vi "Create.vi"(8 "error in (no error)":errorcluster, 10 "Input":string) -> (0 "error out":errorcluster, 3 "Proto":refnum<class "NetAn.lvclass">)   [LabVIEW 2020, in "NetAn.lvclass"]
uses:
  NetAn.lvclass
  <vilib>/Utility/miscctls.llb/LVMapReplaceAction.ctl
  NetAn.lvclass/NetAn.ctl
  Global 1.vi
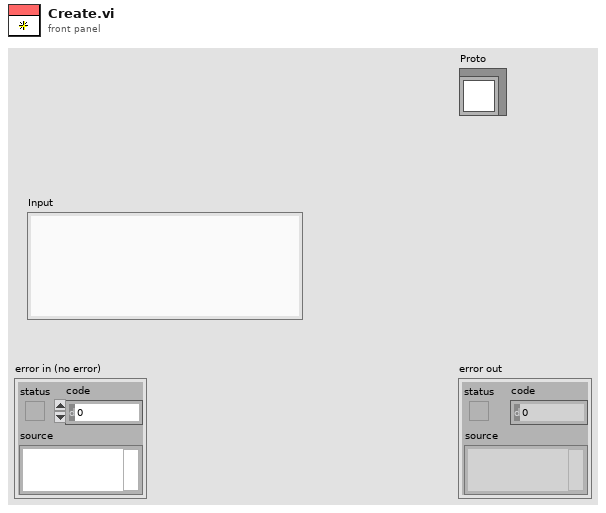
[diagram p1: front panel]
types:
  T1 = typedef "LVMapReplaceAction.ctl" = enum32{"Modify Entry only if found", "Add or Modify Entry", "Delete Entry"}
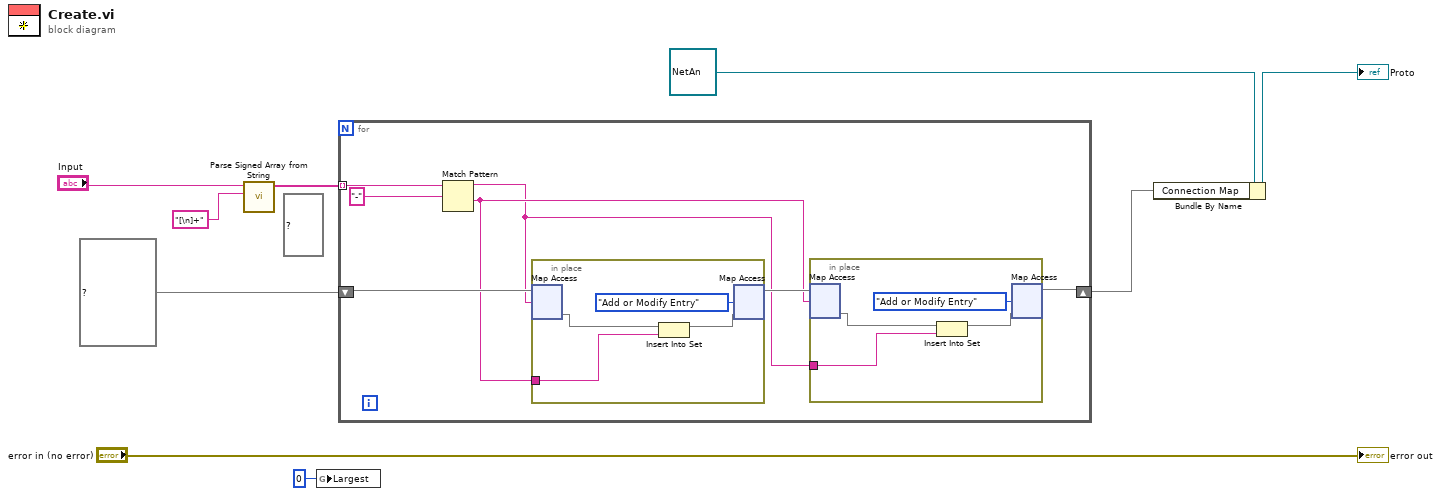
[diagram p0: block diagram]
diagram:
  (unwired) set{string} {} ("set in")
  n1 = call "Parse Signed Array from String.vi"("Delimiter regex"="[\n]+", "Input"="Input") -> ("Parsed Array"=w4:string[])  [unwired: 8 in, 1 out]
  n2 = global write "Global 1.vi" "Largest"(0 ("Largest")) -> ()
  n3 = for {
    tunnel: w4 -> [w16] mode=indexing
    shift-right: [w12] -> w2
    shift-left: map{string, set{string}} {} ("map") -> [w14]
    n4 = Match Pattern(string=w16, regular expression="-") -> (before substring=w10:string, after substring=w11:string)  [unwired: 1 in, 2 out]
    n5 = in-place {
      in-place-border: w11 -> [w22]
      n6 = in-place-map #1(w14, w10) -> (w24:set{string})  [unwired: 1 in, 1 out]
      n7 = Insert Into Set(10:w22, 11:w24) -> (3:w23:set{string})  [unwired: 1 out]
      n8 = in-place-map #1(w23, LVMapReplaceAction."Add or Modify Entry" ("action")) -> (w13:map{string, set{string}})  [unwired: 2 out]
    }
    n9 = in-place {
      in-place-border: w10 -> [w18]
      n10 = in-place-map #2(w13, w11) -> (w20:set{string})  [unwired: 1 in, 1 out]
      n11 = Insert Into Set(10:w18, 11:w20) -> (3:w19:set{string})  [unwired: 1 out]
      n12 = in-place-map #2(w19, LVMapReplaceAction."Add or Modify Entry" ("action")) -> (w12:map{string, set{string}})  [unwired: 2 out]
    }
  }
  n13 = Bundle By Name(cluster=refnum<class "NetAn.lvclass"> refnum ("Proto"), "Connection Map"=w2) -> (→"Proto":refnum<class "NetAn.lvclass">)
  "error out" <- "error in (no error)"
